vi "synnax channel retrieve keys Single.vi"(0 "client":u64, 5 "name":string, 11 "error in (no error)":errorcluster) -> (4 "client out":u64, 6 "key":u32, 15 "error out":errorcluster)   [LabVIEW 2026, in "synnax_clib.lvlib"]
doc: "SYNNAX_EXPORT int32_t synnax_channel_retrieve_keys(\n SynnaxClient client,\n const char **names,\n uint64_t name_count,\n uint32_t *out_keys,\n SynnaxError err\n);"
uses:
  synnax_clib.lvlib
  synnax_clib.dll
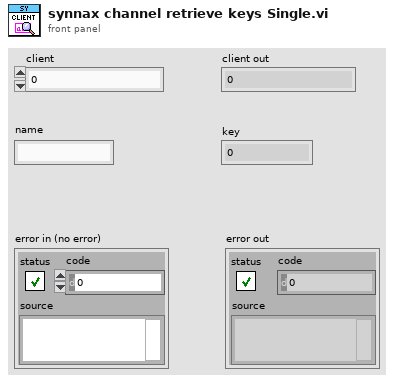
[diagram p1: front panel]
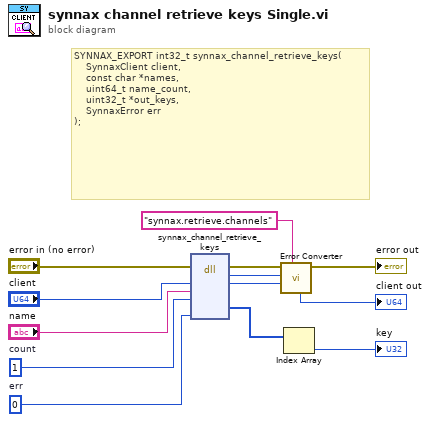
[diagram p0: block diagram]
diagram:
  w2 = u64 1  # count
  w5 = u64 0  # err
  # "SYNNAX_EXPORT int32_t synnax_channel_retrieve_keys(\n    SynnaxClient client,\n    const char *names,\n    uint64_t name_count,\n    uint32_t *out_keys,\n    SynnaxError err\n);"
  n1 = dll-call lib="C/synnax/client/labview/synnax_clib.*" fn="synnax_channel_retrieve_keys"(error in="error in (no error)", "client"="client", "names"="name", "name_count"=w2, "err"=w5) -> (error out=w7:errorcluster, "return type"=w9:i32, "client"=→"client out":u64, "out_keys"=w4:u32[])  [unwired: 6 in, 1 out]
  n2 = call "Error Converter.vi"("source"="synnax.retrieve.channels", "error code"=w9, "error in (no error)"=w7) -> ("error out"=→"error out":errorcluster)  [unwired: 8 in]
  n3 = Index Array(array=w4) -> (element=→"key":u32)  [unwired: 1 in]
